vi "Motor (1).vi"() -> ()   [LabVIEW 2020]
doc: "Manually blink and LED attached to a digital output channel of a LINX device by clicking and LED control in LabVIEW."
uses:
  <vilib>/MakerHub/LINX/Public/Peripherals/PWM/PWM Set Duty Cycle 1 Chan.vi
  <vilib>/MakerHub/LINX/Public/Peripherals/Digital/Digital Write 1 Chan.vi
  <vilib>/MakerHub/LINX/Public/Peripherals/Digital/Digital Write N Chans.vi
  <vilib>/MakerHub/LINX/Private/Local IO/LinxDigitalWrite.vi
  <vilib>/MakerHub/LINX/Public/Utilities/Check Channel.vi
  <vilib>/MakerHub/LINX/Public/Utilities/Open Serial.vi
  <userlib>/_OpenG.lib/comparison/comparison.llb/Boolean Changed__ogtk.vi
  <vilib>/MakerHub/LINX/Public/Peripherals/PWM/PWM Set Duty Cycle N Chans.vi
  <vilib>/MakerHub/LINX/Private/Utilties/Generate Error.vi
  <vilib>/MakerHub/LINX/LMH-LINX.lvlib
panel:
  in  "DIRECTION":bool
  in  "AI Channel":u8
  in  "In 2":u8=4
  in  "In 1":u8=3
  in  "MOTOR Channel":u8=5
  out "Loop Rate (Hz)":u32=69
  out "PWM Out (0-1)":dbl(knob) scale=0.0..1.0 scale format="%.2f"
  in  "LED Channel":u8=9
  in  "Serial Port":refnum<visa-resource-name>="COM9"
  in  "Stop Button":bool
  # "This example was created by combining code from LINX - Blink (Simple), LINX - PWM 1 Channel, and LINX - Photocell VIs\nIn addition, the circuitry for how to control a DC motor was modified from the example in:\nElegoo The Most Complete Starter Kit for UNO V2.0.2020.4.3\\English\\Part 2 Module Learning\\2.23 DC Motors"
  # "LINX Device Settings"
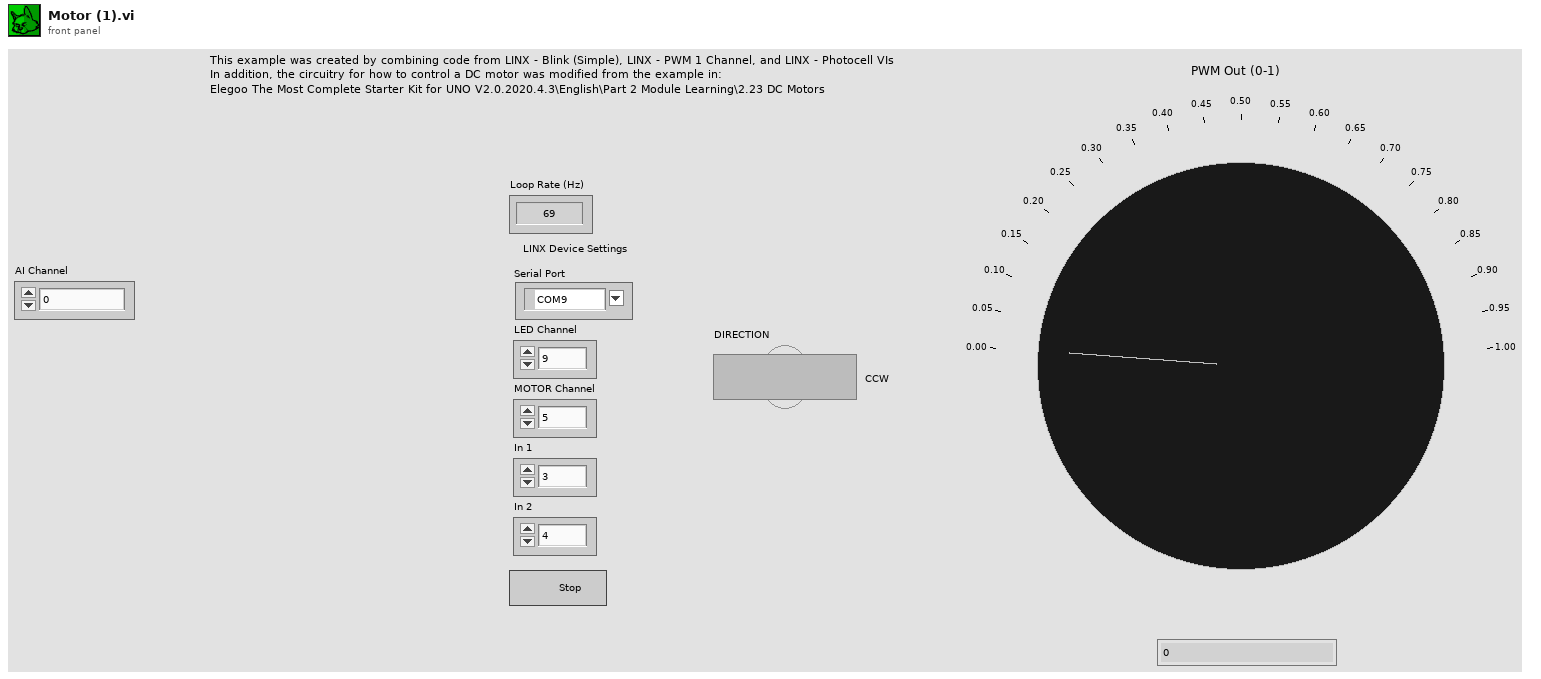
[diagram p1: front panel]
types:
  T1 = typedef "LMH-LINX.lvlib/LINX Ref.ctl" = cluster{"IO":T2, "Interface":T3, "LINX Device Config":T4}
  T2 = typedef "LMH-LINX.lvlib/Platform.ctl" = enum16{"Remote", "Local"}
  T3 = typedef "LMH-LINX.lvlib/Interface.ctl" = enum16{"Serial", "TCP"}
  T4 = typedef "LMH-LINX.lvlib/Device.lvlib/LINX Device Config.ctl" = cluster{"Interface":T3, "COM Port":refnum<visa-resource-name>, "TCP Configuration":T5, "Device Family":u8, "Device ID":u8, "Device Name":string, "TCP Ref":refnum<k5>, "Channels":T6}
  T5 = typedef "LMH-LINX.lvlib/Device.lvlib/TCP Config.ctl" = cluster{"IP Address":string, "Port":u16}
  T6 = typedef "LMH-LINX.lvlib/Channels.ctl" = cluster{"DI":u8[], "DO":u8[], "AI":u8[], "AO":u8[], "PWM":u8[], "QE":u8[], "UART":u8[], "I2C 2":u8[], "SPI":u8[], "CAN":u8[], "Servo":u8[], "AI Ref (V)":dbl, "AI Resolution (Bits)":u8, "AO Ref (V)":dbl, "AO Resolution (Bits)":u8}
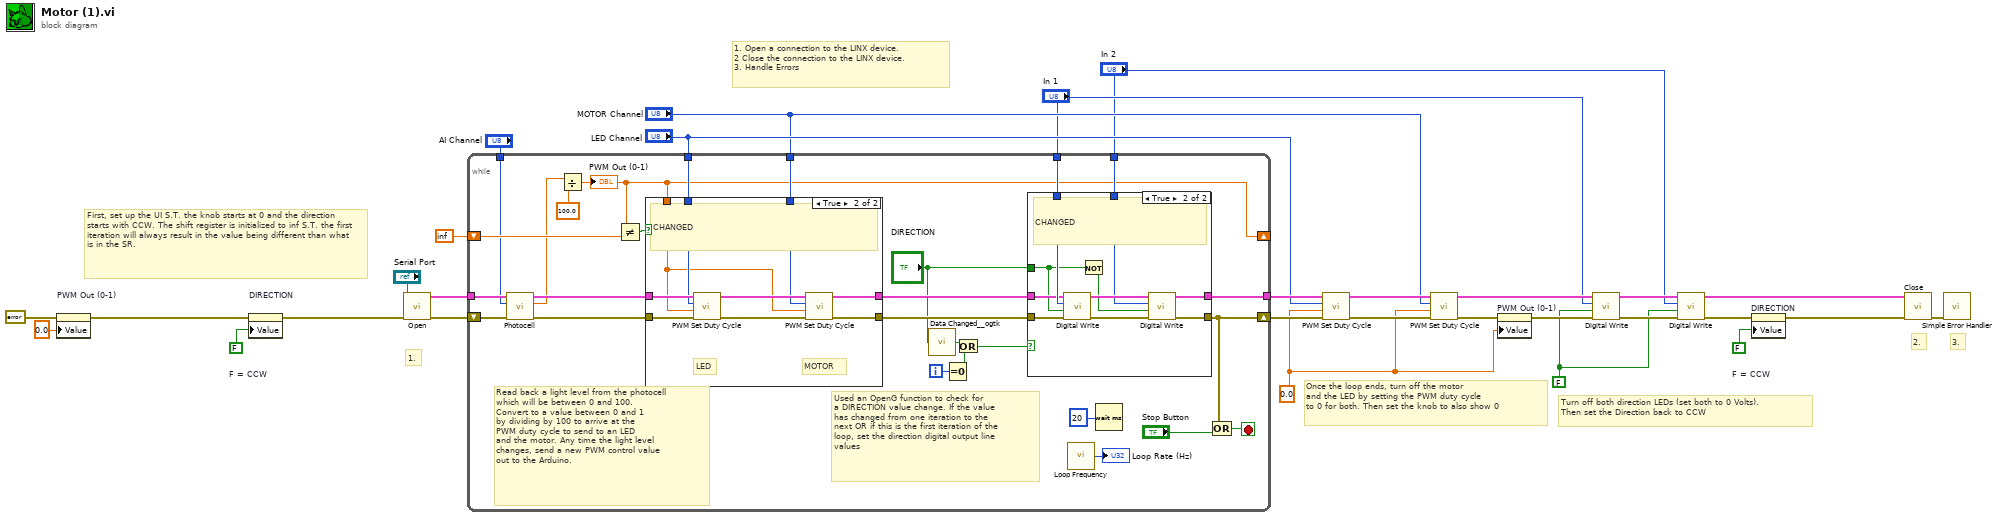
[diagram p0: block diagram]
diagram:
  w3 = FALSE  # F = CCW
  w4 = FALSE  # F = CCW
  w8 = FALSE
  w16 = 0.0
  # "Turn off both direction LEDs (set both to 0 Volts).\nThen set the Direction back to CCW"
  # "Once the loop ends, turn off the motor\nand the LED by setting the PWM duty cycle\nto 0 for both. Then set the knob to also show 0"
  # "First, set up the UI S.T. the knob starts at 0 and the direction starts with CCW. The shift register is initialized to inf S.T. the first iteration will always result in the value being different than what is in the SR."
  # "1. Open a connection to the LINX device.\n2 Close the connection to the LINX device.\n3. Handle Errors"
  # "3."
  # "2."
  # "1."
  n1 = property on="PWM Out (0-1)" class="Knob (strict)"(error in=errorcluster {"status"=FALSE, "code"=0, "source"=""} ("Error In"), "Value"=0.0) -> (error out=w6:errorcluster)  [unwired: 1 in, 1 out]
  n2 = property on="DIRECTION" class="Bool (strict)"(error in=w6, "Value"=w4) -> (error out=w5:errorcluster)  [unwired: 1 in, 1 out]
  n3 = call-poly <vilib>:"Open.vi"("Error In"=w5, "Serial Port"="Serial Port") -> ("Error Out"=w29:errorcluster, "LINX Resource"=w30:T1)  [unwired: 7 in, 1 out]
  n4 = while {
    tunnel: w30 -> [w41]
    tunnel: [w46] -> w22
    shift-right: [w45] -> w23
    shift-left: w29 -> [w43]
    tunnel: "LED Channel" -> [w54]
    shift-right: [w36] -> _
    shift-left: inf -> [w53]
    tunnel: "MOTOR Channel" -> [w50]
    tunnel: "In 1" -> [w49]
    tunnel: "In 2" -> [w44]
    tunnel: "AI Channel" -> [w40]
    i -> [w34]
    stop <- w57 stop-if-true
    # "Used an OpenG function to check for\na DIRECTION value change. If the value\nhas changed from one iteration to the\nnext OR if this is the first iteration of the\nloop, set the direction digital output line\nvalues"
    # "Read back a light level from the photocell\nwhich will be between 0 and 100.\nConvert to a value between 0 and 1\nby dividing by 100 to arrive at the\nPWM duty cycle to send to an LED\nand the motor. Any time the light level\nchanges, send a new PWM control value\nout to the Arduino."
    n5 = call <vilib>:"Photocell.vi"("Error In"=w43, "AI Channel"=w40, "LINX Resource"=w41) -> ("Error Out"=w42:errorcluster, "Value (0-100)"=w38:dbl, "LINX Resource"=w39:T1)  [unwired: 6 in]
    n6 = Divide(x=w38, y=100.0) -> (x/y=w36:dbl)
    "PWM Out (0-1)" <- w36
    n7 = Not Equal?(x=w36, y=w53) -> (x != y?=w52:bool)
    n8 = case shown="True" w52 {
      tunnel: w39 -> [w59 w68]
      tunnel: [w59 w64] -> w48
      tunnel: w42 -> [w58 w67]
      tunnel: [w58 w62] -> w47
      tunnel: w36 -> [_ w60]
      tunnel: w54 -> [_ w66]
      tunnel: w50 -> [_ w61]
      frame False {
        # "SAME"
      }
      frame True {
        # "MOTOR"
        # "LED"
        # "CHANGED"
        n9 = call-poly <vilib>:"PWM Set Duty Cycle.vi"("Error In"=w67, "Duty Cycle (0-1)"=w60, "PWM Channel"=w66, "LINX Resource"=w68) -> ("Error Out"=w63:errorcluster, "LINX Resource"=w65:T1)  [unwired: 6 in]
        n10 = call-poly <vilib>:"PWM Set Duty Cycle.vi"("Error In"=w63, "Duty Cycle (0-1)"=w60, "PWM Channel"=w61, "LINX Resource"=w65) -> ("Error Out"=w62:errorcluster, "LINX Resource"=w64:T1)  [unwired: 6 in]
      }
    }
    n11 = call-poly <userlib>:"Data Changed__ogtk.vi"("Boolean"="DIRECTION") -> ("Changed"=w31:bool)
    n12 = Equal To 0?(x=w34) -> (x = 0?=w33:bool)
    n13 = Or(x=w31, y=w33) -> (x .or. y?=w32:bool)
    n14 = case shown="True" w32 {
      tunnel: "DIRECTION" -> [_ w72]
      tunnel: w49 -> [_ w80]
      tunnel: w48 -> [w70 w79]
      tunnel: w47 -> [w69 w78]
      tunnel: [w70 w75] -> w46
      tunnel: [w69 w74] -> w45
      tunnel: w44 -> [_ w73]
      frame False {
        # "SAME"
      }
      frame True {
        # "CHANGED"
        n15 = call-poly <vilib>:"Digital Write.vi"("Error In"=w78, "Output Value"=w72, "DO Channel"=w80, "LINX Resource"=w79) -> ("Error Out"=w77:errorcluster, "LINX Resource"=w76:T1)  [unwired: 6 in]
        n16 = Not(x=w72) -> (.not. x?=w71:bool)
        n17 = call-poly <vilib>:"Digital Write.vi"("Error In"=w77, "Output Value"=w71, "DO Channel"=w73, "LINX Resource"=w76) -> ("Error Out"=w74:errorcluster, "LINX Resource"=w75:T1)  [unwired: 6 in]
      }
    }
    n18 = call <vilib>:"Loop Frequency.vi"() -> ("Loop Rate (Hz)"=→"Loop Rate (Hz)":u32)
    n19 = Wait (ms)(milliseconds to wait=u32 20) -> ()  [unwired: 1 out]
    n20 = Or(x=w45, y="Stop Button") -> (x .or. y?=w57:bool)
  }
  n21 = call-poly <vilib>:"PWM Set Duty Cycle.vi"("Error In"=w23, "Duty Cycle (0-1)"=w16, "PWM Channel"="LED Channel", "LINX Resource"=w22) -> ("Error Out"=w19:errorcluster, "LINX Resource"=w20:T1)  [unwired: 6 in]
  n22 = call-poly <vilib>:"PWM Set Duty Cycle.vi"("Error In"=w19, "Duty Cycle (0-1)"=w16, "PWM Channel"="MOTOR Channel", "LINX Resource"=w20) -> ("Error Out"=w18:errorcluster, "LINX Resource"=w15:T1)  [unwired: 6 in]
  n23 = property on="PWM Out (0-1)" class="Knob (strict)"(error in=w18, "Value"=w16) -> (error out=w11:errorcluster)  [unwired: 1 in, 1 out]
  n24 = call-poly <vilib>:"Digital Write.vi"("Error In"=w11, "Output Value"=w8, "DO Channel"="In 1", "LINX Resource"=w15) -> ("Error Out"=w12:errorcluster, "LINX Resource"=w14:T1)  [unwired: 6 in]
  n25 = call-poly <vilib>:"Digital Write.vi"("Error In"=w12, "Output Value"=w8, "DO Channel"="In 2", "LINX Resource"=w14) -> ("Error Out"=w2:errorcluster, "LINX Resource"=w13:T1)  [unwired: 6 in]
  n26 = property on="DIRECTION" class="Bool (strict)"(error in=w2, "Value"=w3) -> (error out=w1:errorcluster)  [unwired: 1 in, 1 out]
  n27 = call <vilib>:"Close.vi"("Error In"=w1, "LINX Resource"=w13) -> ("Error Out"=w27:errorcluster)  [unwired: 9 in]
  n28 = call <vilib>:"Simple Error Handler.vi"("error in (no error)"=w27) -> ()  [unwired: 4 in, 5 out]
